vi "Get Attribute VAR.vi"(8 "error in":errorcluster, 10 "Attribute":string, 11 "ConfigFromJSON in":refnum<class "Config Hardcoded.lvclass">) -> (0 "error out":errorcluster, 2 "Value":variant, 3 "ConfigFromJSON out":refnum<class "Config Hardcoded.lvclass">)   [LabVIEW 2024, in "PCAN.lvlib" / "Config Hardcoded.lvclass"]
uses:
  Config Hardcoded.lvclass
  Config Hardcoded.lvclass/Config Hardcoded.ctl
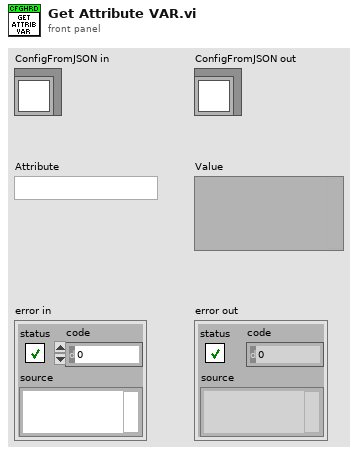
[diagram p1: front panel]
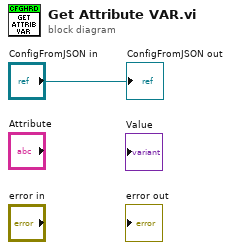
[diagram p0: block diagram]
diagram:
  "ConfigFromJSON out" <- "ConfigFromJSON in"
